vi "Move.vi"(8 "error in (no error)":errorcluster, 10 "Amount (rev)":dbl, 11 "AlphaStep One in":refnum<class "AlphaStep One.lvclass">) -> (0 "error out":errorcluster, 3 "AlphaStep One out":refnum<class "AlphaStep One.lvclass">)   [LabVIEW 2015, in "AlphaStep One.lvclass"]
uses:
  AlphaStep One.lvclass
  AlphaStep One.lvclass/AlphaStep One.ctl
  Serial Device/Serial Device.lvclass
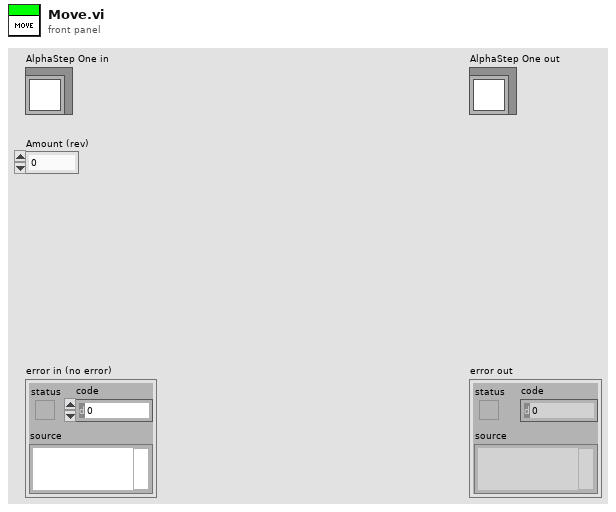
[diagram p1: front panel]
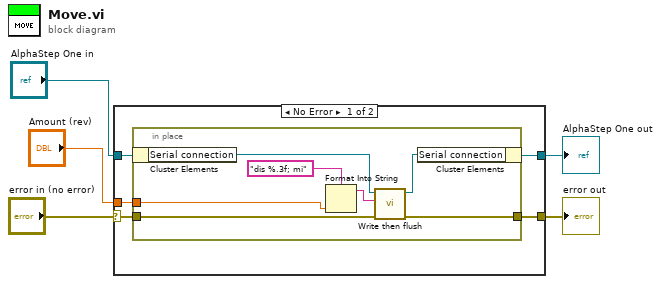
[diagram p0: block diagram]
diagram:
  n1 = case shown="No Error" "error in (no error)" {
    selector: "error in (no error)" -> [w9 w19]
    tunnel: [w8 w19] -> w4
    tunnel: "AlphaStep One in" -> [w7 w18]
    tunnel: "Amount (rev)" -> [w10 _]
    tunnel: [w6 w18] -> w1
    frame No Error {
      n2 = in-place {
        in-place-border: w10 -> [w17]
        in-place-border: w9 -> [w15]
        in-place-border: [w14] -> w8
        n3 = in-place-cluster #1(w7) -> ("Serial connection"=w13:refnum<class "Serial Device.lvclass">)
        n4 = Format Into String(format string="dis %.3f; mi", w17) -> (resulting string=w16:string)  [unwired: 2 in, 1 out]
        n5 = call "Write then flush.vi"("error in (no error)"=w15, "TX Data"=w16, "Serial Device in"=w13) -> ("error out"=w14:errorcluster, "Serial Device out"=w12:refnum<class "Serial Device.lvclass">)  [unwired: 7 in]
        n6 = in-place-cluster #1("Serial connection"=w12) -> (w6:refnum<class "AlphaStep One.lvclass">)
      }
    }
    frame Error {
    }
  }
  "error out" <- w4
  "AlphaStep One out" <- w1
